vi "prime_lines_media.vi"(8 "error in (no error)":errorcluster, 11 "GLOBAL SETTINGS IN":refnum<notifier>) -> (0 "error out":errorcluster, 3 "GLOBAL SETTINGS OUT":refnum<notifier>)   [LabVIEW 2013]
uses:
  main_machine/type_defs/global_settings.ctl
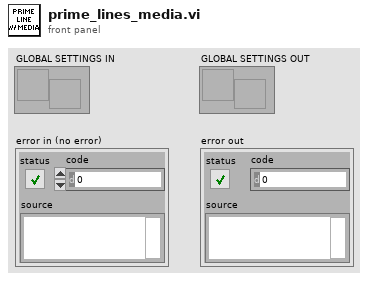
[diagram p1: front panel]
types:
  T1 = typedef "global_settings.ctl" = cluster{"# REACTORS":u32, "17X PORT":i32, "WASTE POSITION ":i32, "SECONDS BETWEEN SAMPLING":dbl, "FACS DIVA DIRECTORY":path, "DATA FILE":path, "REACTORS TO USE":u32[], "PULSE PERIOD":i32, "USE LIGHTS?":bool, "LED FILE":path, "LED CHANNELS":u32[], "PULSE LENGTH":i32, "SUMMARY FILE":path, "OUTGROWTH TIME POINTS":dbl, "SELECTION VALVE PORT":refnum<visa-resource-name>, "HTS PORT":refnum<visa-resource-name>, "DILUTION VOLUME (uL)":i32, "DILUTION FILE":path, "1X PORT":i32}
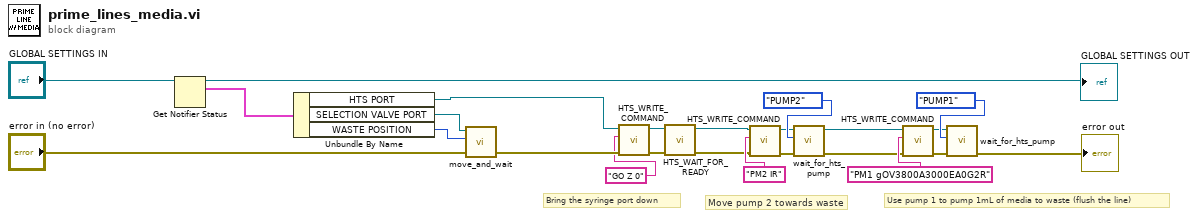
[diagram p0: block diagram]
diagram:
  # "Bring the syringe port down"
  # "Use pump 1 to pump 1mL of media to waste (flush the line)"
  # "Move pump 2 towards waste"
  n1 = Get Notifier Status(notifier="GLOBAL SETTINGS IN") -> (notifier out=→"GLOBAL SETTINGS OUT":refnum<notifier>, current notification=w22:T1)  [unwired: 1 in, 3 out]
  n2 = Unbundle By Name(w22) -> ("HTS PORT"=w23:refnum<visa-resource-name>, "SELECTION VALVE PORT"=w16:refnum<visa-resource-name>, "WASTE POSITION"=w17:i32)
  n3 = call "move_and_wait.vi"("Error IN"="error in (no error)", "MOVE TO POSITION"=w17, "VISA Resource IN"=w16) -> ("Error OUT"=w19:errorcluster)  [unwired: 6 in, 2 out]
  n4 = call "HTS_WRITE_COMMAND.vi"("Error IN"=w19, "Command"="GO Z 0", "HTS PORT IN"=w23) -> ("Error OUT"=w15:errorcluster, "HTS PORT OUT"=w14:refnum<visa-resource-name>)  [unwired: 6 in, 1 out]
  n5 = call "HTS_WAIT_FOR_READY.vi"("Error IN"=w15, "VISA resource IN"=w14) -> ("Error OUT"=w3:errorcluster, "VISA resource OUT"=w4:refnum<visa-resource-name>)  [unwired: 6 in, 2 out]
  n6 = call "HTS_WRITE_COMMAND.vi"("Error IN"=w3, "Command"="PM2 IR", "HTS PORT IN"=w4) -> ("Error OUT"=w7:errorcluster, "HTS PORT OUT"=w6:refnum<visa-resource-name>)  [unwired: 6 in, 1 out]
  n7 = call "wait_for_hts_pump.vi"("error in (no error)"=w7, "PUMP"=enum16{"PUMP2", "PUMP1"}."PUMP2", "HTS PORT IN"=w6) -> ("error out"=w1:errorcluster, "HTS PORT OUT"=w2:refnum<visa-resource-name>)  [unwired: 7 in]
  n8 = call "HTS_WRITE_COMMAND.vi"("Error IN"=w1, "Command"="PM1 gOV3800A3000EA0G2R", "HTS PORT IN"=w2) -> ("Error OUT"=w11:errorcluster, "HTS PORT OUT"=w10:refnum<visa-resource-name>)  [unwired: 6 in, 1 out]
  n9 = call "wait_for_hts_pump.vi"("error in (no error)"=w11, "PUMP"=enum16{"PUMP2", "PUMP1"}."PUMP1", "HTS PORT IN"=w10) -> ("error out"=→"error out":errorcluster)  [unwired: 7 in, 1 out]
